vi "Practica5_Servo.vi"() -> ()   [LabVIEW 2015]
uses:
  <vilib>/LabVIEW Interface for Arduino/LabVIEW Interface for Arduino.lvlib
panel:
  in  "Velocidad":u8(knob) scale=0.0..10.0
  in  "stop":bool
  in  "Angulo":u8(knob) scale=0.0..180.0
  out "Meter":u8(knob) scale=0.0..180.0
  # "Control de Servo"
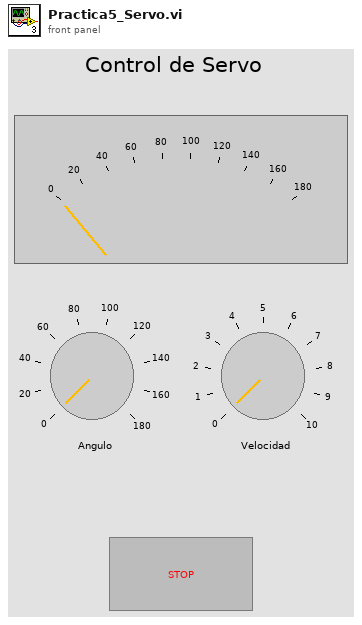
[diagram p1: front panel]
types:
  T1 = typedef "LabVIEW Interface for Arduino.lvlib/Arduino Resource.ctl" = cluster{"VISA resource":refnum<visa-resource-name>, "Board Type":T2, "Connection Type":enum8{"USB / Serial"}, "Bytes Per Packet (15)":u8}
  T2 = typedef "LabVIEW Interface for Arduino.lvlib/Board Type.ctl" = enum16{"Uno", "Dimuelanove w/Atmega 328", "Mega 2560"}
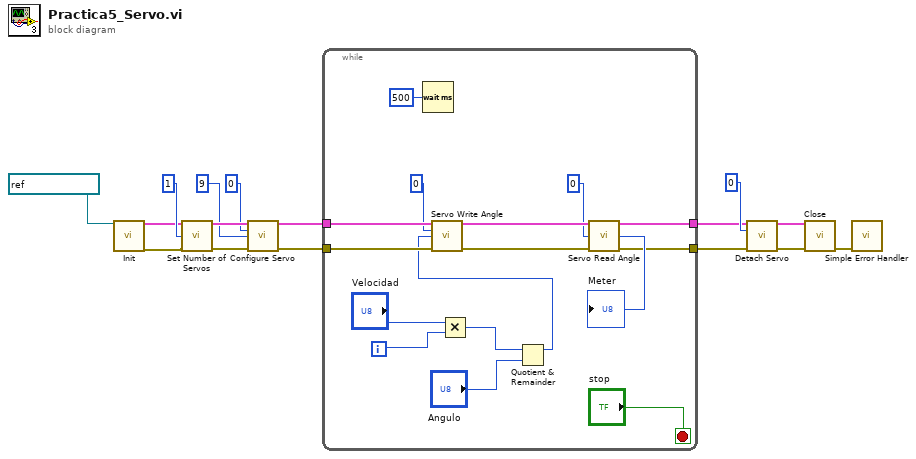
[diagram p0: block diagram]
diagram:
  n1 = call <vilib>:"Init.vi"("VISA resource"=refnum<visa-resource-name> "COM3") -> ("Arduino Resource"=w14:T1, "error out"=w13:errorcluster)  [unwired: 17 in]
  n2 = call <vilib>:"Set Number of Servos.vi"("Arduino Resource"=w14, "Number Of Servos (1)"=u8 1, "error in"=w13) -> ("Arduino Resource"=w12:T1, "error out"=w11:errorcluster)  [unwired: 11 in]
  n3 = call <vilib>:"Configure Servo.vi"("Arduino Resource"=w12, "Servo Number (0)"=u8 0, "DIO Pin (2)"=u8 9, "error in"=w11) -> ("Arduino Resource"=w9:T1, "error out"=w10:errorcluster)  [unwired: 10 in]
  n4 = while {
    tunnel: w10 -> [w32]
    tunnel: w9 -> [w31]
    tunnel: [w24] -> w2
    tunnel: [w23] -> w1
    i -> [w22]
    stop <- "stop" stop-if-true
    n5 = Wait (ms)(milliseconds to wait=u32 500) -> ()  [unwired: 1 out]
    n6 = Multiply(x="Velocidad", y=w22) -> (x*y=w19:i32)
    n7 = Quotient & Remainder(x=w19, y="Angulo") -> (x-y*floor(x/y)=w18:i32)  [unwired: 1 out]
    n8 = call <vilib>:"Servo Write Angle.vi"("Arduino Resource"=w31, "Servo Number"=u8 0, "Angle (Degrees)"=w18, "error in"=w32) -> ("Arduino Resource"=w28:T1, "error out"=w27:errorcluster)  [unwired: 10 in]
    n9 = call <vilib>:"Servo Read Angle.vi"("Arduino Resource"=w28, "Servo Number"=u8 0, "error in"=w27) -> ("Arduino Resource"=w24:T1, "Angle (Degrees)"=→"Meter":u8, "error out"=w23:errorcluster)  [unwired: 10 in]
  }
  n10 = call <vilib>:"Detach Servo.vi"("Arduino Resource"=w2, "Servo Number"=u8 0, "error in"=w1) -> ("Arduino Resource"=w6:T1, "error out"=w5:errorcluster)  [unwired: 11 in]
  n11 = call <vilib>:"Close.vi"("Arduino Resource"=w6, "error in"=w5) -> ("error out"=w4:errorcluster)  [unwired: 13 in]
  n12 = call <vilib>:"Simple Error Handler.vi"("error in (no error)"=w4) -> ()  [unwired: 4 in, 5 out]
